vi "TBQ_Reset.vi"(11 "TimeBasedQueue In":refnum<class "TimeBasedQueue.lvclass">) -> (3 "TimeBasedQueue Out":refnum<class "TimeBasedQueue.lvclass">)   [LabVIEW 2012, in "TimeBasedQueue.lvclass"]
uses:
  TimeBasedQueue.lvclass
  TimeBasedQueue.lvclass/TimeBasedQueue.ctl
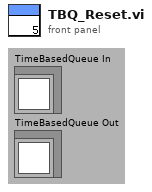
[diagram p1: front panel]
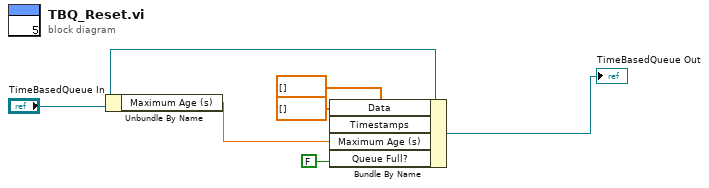
[diagram p0: block diagram]
diagram:
  n1 = Unbundle By Name("TimeBasedQueue In") -> ("Maximum Age (s)"=w5:dbl)
  n2 = Bundle By Name(cluster="TimeBasedQueue In", "Data"=dbl[] [], "Timestamps"=dbl[] [], "Maximum Age (s)"=w5, "Queue Full?"=FALSE) -> (→"TimeBasedQueue Out":refnum<class "TimeBasedQueue.lvclass">)
